vi "Add Implementations to Tree.vi"(8 "error in (no error)":errorcluster, 9 "Wired-in Class Refnum":refnum<vi>, 10 "Method Name":string, 11 "Tree Refnum":refnum<vi>) -> (0 "error out":errorcluster, 2 "Tree Refnum out":refnum<vi>, 3 "All Classes":refnum<vi>[](array[refnum]), 5 "Implementor Lookup":map{string, string}(c390))   [LabVIEW 2020, in "Peek Window.lvlib"]
uses:
  Peek Window.lvlib
  Implementor Tree Item Info.ctl
  Symbols Enum.ctl
  b7fde728-2108-4602-8341-146d6e5bbae3.vi
  <vilib>/Comparison/Equal/Equal Functor/Equal Functor.lvclass
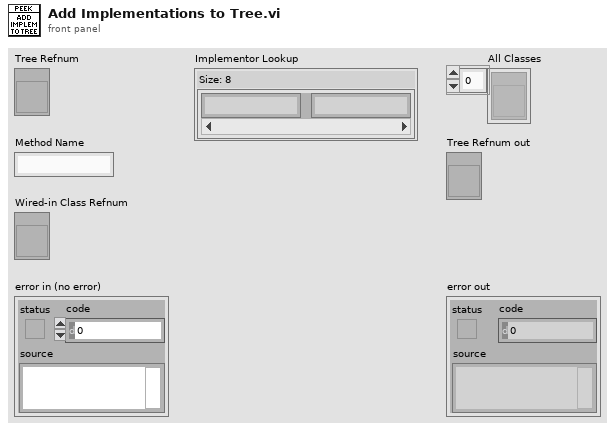
[diagram p1: front panel]
types:
  T1 = typedef "Peek Window.lvlib/Symbols Enum.ctl" = enum16{"<Blank>", "Below Here Glyph", "VI", "Dynamic Dispatch VI"}
  T2 = typedef "Peek Window.lvlib/Implementor Tree Item Info.ctl" = cluster{"ClassRef":refnum<vi>, "Implementor?":bool, "Parent ItemID":string, "Full Qualified Name":string}
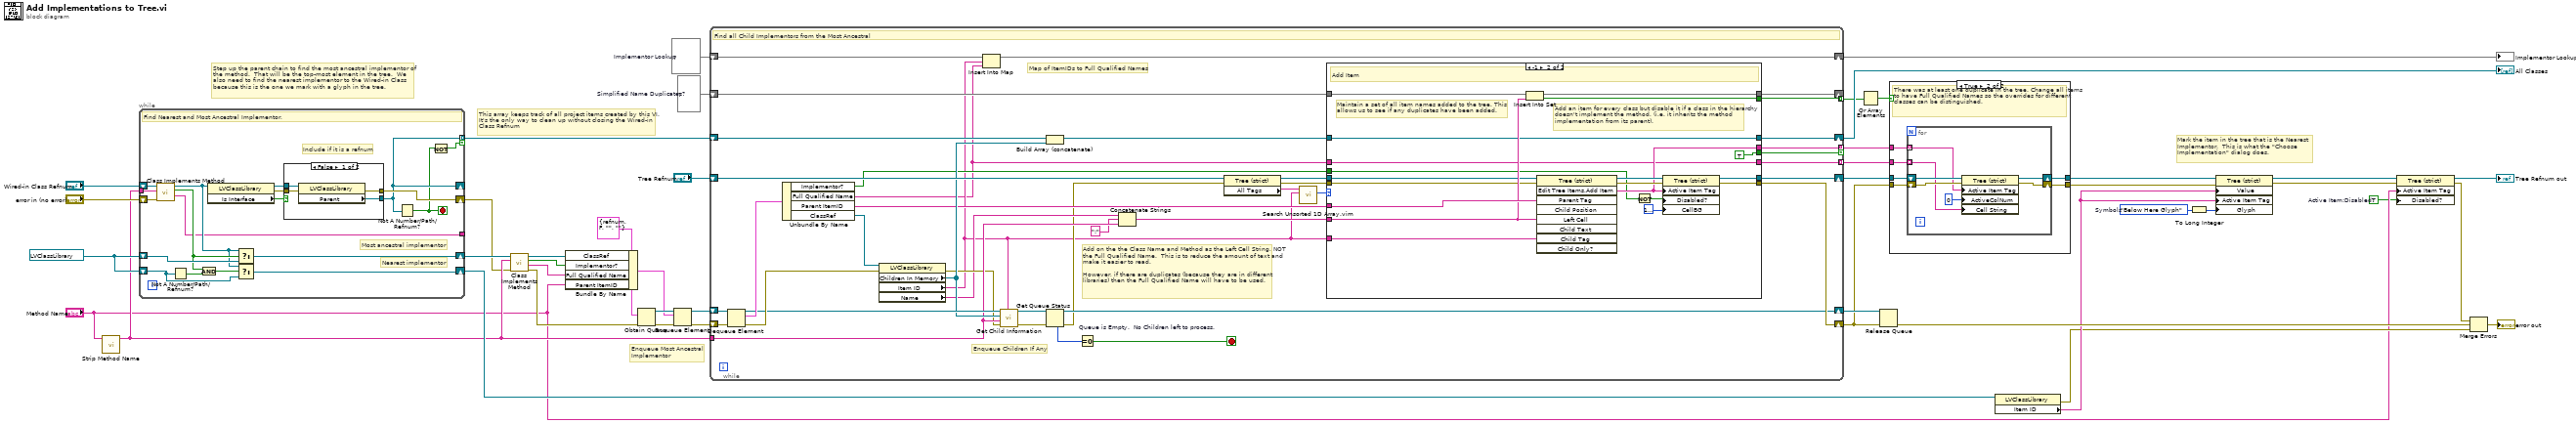
[diagram p0: block diagram]
diagram:
  w3 = TRUE  # Active Item:Disabled?
  w19 = Symbols_Enum."Below Here Glyph"  # Symbols
  w20 = set{string} {}  # Simplified Name Duplicates?
  w23 = map{string, string} {}  # Implementor Lookup
  w35 = refnum<vi> refnum ("Class Refnum out")
  w39 = T2 {"ClassRef"=refnum, "Implementor?"=FALSE, "Parent ItemID"="", "Full Qualified Name"=""} ("Cluster")
  # "Mark the item in the tree that is the Nearest Implementor.  This is what the \"Choose Implementation\" dialog does."
  # "Enqueue Most Ancestral\nImplementor"
  # "This array keeps track of all project items created by this VI.\nIt's the only way to clean up without closing the Wired-in \nClass Refnum"
  # "Step up the parent chain to find the most ancestral implementor of\nthe method.  That will be the top-most element in the tree.  We\nalso need to find the nearest implementor to the Wired-in Class\nbecause this is the one we mark with a glyph in the tree."
  n1 = call "Strip Method Name.vi"("Full Qualified Name in"="Method Name") -> ("Plain Method Name out"=w21:string)  [unwired: 10 in]
  n2 = while {
    shift-right: [w59] -> w24
    shift-left: w35 -> [w60]
    shift-right: [w47] -> _
    shift-left: "Wired-in Class Refnum" -> [w62]
    shift-right: [w53] -> w13
    shift-left: "error in (no error)" -> [w63]
    tunnel: w21 -> [w61]
    shift-right: [w54] -> w36
    shift-left: w35 -> [w55]
    tunnel: [w48] -> _
    tunnel: [w47] -> w25 mode=indexing if=w45
    stop <- w46 stop-if-true
    # "Include if it is a refnum"
    # "Nearest implementor"
    # "Most ancestral implementor"
    # "Find Nearest and Most Ancestral Implementor,"
    n3 = call "Class Implements Method.vi"("error in (no error)"=w63, "Method Name"=w61, "Class Refnum"=w62) -> ("VI Qualified Name"=w48:string, "Implements method?"=w57:bool, "Class Refnum out"=w50:refnum<vi>)  [unwired: 5 in, 1 out]
    n4 = Not A Number/Path/Refnum?(number/path/refnum=w55) -> (NaN/Path/Refnum?=w58:bool)
    n5 = And(x=w57, y=w58) -> (x .and. y?=w56:bool)
    n6 = property class="LVClassLibrary"(reference=w50) -> (reference out=w52:refnum<vi>, error out=w51:errorcluster, "Is Interface"=w49:bool)  [unwired: 1 in]
    n7 = Select(t=w50, s=w57, f=w60) -> (s? t:f=w59:refnum<vi>)
    n8 = Select(t=w50, s=w56, f=w55) -> (s? t:f=w54:refnum<vi>)
    n9 = case shown="False" w49 {
      tunnel: [w67 w68] -> w53
      tunnel: [w66 _] -> w47
      tunnel: w52 -> [w65 _]
      tunnel: w51 -> [w64 w68]
      frame False {
        n10 = property class="LVClassLibrary"(reference=w65, error in=w64) -> (error out=w67:errorcluster, "Parent"=w66:refnum<vi>)  [unwired: 1 out]
      }
      frame True {
      }
    }
    n11 = Not A Number/Path/Refnum?(number/path/refnum=w47) -> (NaN/Path/Refnum?=w46:bool)
    n12 = Not(x=w46) -> (.not. x?=w45:bool)
  }
  n13 = call "Class Implements Method.vi"("error in (no error)"=w13, "Method Name"=w21, "Class Refnum"=w24) -> ("error out"=w12:errorcluster, "VI Qualified Name"=w11:string, "Implements method?"=w10:bool, "Class Refnum out"=w7:refnum<vi>)  [unwired: 5 in]
  n14 = Bundle By Name(cluster=w39, "ClassRef"=w7, "Implementor?"=w10, "Full Qualified Name"=w11, "Parent ItemID"="Method Name") -> (w42:T2)
  n15 = Obtain Queue(element data type=w39, error in (no error)=w12) -> (queue out=w44:refnum<queue>, error out=w43:errorcluster)  [unwired: 3 in, 1 out]
  n16 = Enqueue Element(queue=w44, element=w42, error in (no error)=w43) -> (queue out=w41:refnum<queue>, error out=w40:errorcluster)  [unwired: 1 in, 1 out]
  n17 = while {
    shift-right: [w99] -> w14
    shift-left: w40 -> [w107]
    tunnel: w21 -> [w94]
    shift-right: [w72] -> w33
    shift-left: w25 -> [w97]
    tunnel: [w95] -> w29 mode=indexing if=w76
    tunnel: [w69] -> w28 mode=indexing
    tunnel: [w84] -> w32 mode=indexing
    shift-right: [w87] -> w22
    shift-left: w23 -> [w88]
    shift-right: [w85] -> _
    shift-left: w20 -> [w86]
    shift-right: [w98] -> w30
    shift-left: "Tree Refnum" -> [w100]
    shift-right: [w92] -> w38
    shift-left: w41 -> [w108]
    stop <- w106 stop-if-true
    # "Add on the the Class Name and Method as the Left Cell String, NOT the Full Qualified Name.  This is to reduce the amount of text and make it easier to read.\n\nHowever, if there are duplicates (because they are in different libraries) then the Full Qualified Name will have to be used."
    # "Enqueue Children If Any"
    # "Map of ItemIDs to Full Qualified Names"
    # "Find all Child Implementors from the Most Ancestral"
    n18 = Dequeue Element(queue=w108, error in (no error)=w107) -> (queue out=w102:refnum<queue>, element=w104:T2, error out=w103:errorcluster)  [unwired: 1 in, 1 out]
    n19 = Unbundle By Name(w104) -> ("Implementor?"=w81:bool, "Full Qualified Name"=w70:string, "Parent ItemID"=w90:string, "ClassRef"=w82:refnum<vi>)
    n20 = property class="LVClassLibrary"(reference=w82, error in=w103) -> (error out=w91:errorcluster, "Children In Memory"=w96:refnum<vi>[], "Item ID"=w74:string, "Name"=w80:string)  [unwired: 1 out]
    n21 = Insert Into Map(map in=w88, key=w74, value=w70) -> (map out=w87:map{string, string})  [unwired: 2 out]
    n22 = call "Get Child Information.vi"("ParentID"=w74, "error in (no error)"=w91, "Plain Method Name in"=w94, "Children in Memory"=w96, "Queue in"=w102) -> ("error out"=w89:errorcluster, "Queue out"=w101:refnum<queue>)  [unwired: 5 in]
    n23 = Build Array (concatenate)(w97, w96) -> (w71:refnum<vi>[])
    n24 = Get Queue Status(queue=w101, error in (no error)=w89) -> (queue out=w92:refnum<queue>, error out=w78:errorcluster, # elements in queue=w105:i32)  [unwired: 1 in, 5 out]
    n25 = Equal To 0? "Queue is Empty.  No Children left to process."(x=w105) -> (x = 0?=w106:bool)
    n26 = Concatenate Strings(w80, ":" ("element"), w94) -> (w83:string)
    n27 = property class="Tree (strict)"(reference=w100, error in=w78) -> (reference out=w79:refnum<vi>, error out=w77:errorcluster, "All Tags"=w75:string[])
    n28 = call "Search Unsorted 1D Array.vim"("element"=w74, "unsorted 1D array"=w75) -> ("index of element"=w73:i32)  [unwired: 9 in]
    n29 = case shown="-1" w73 {
      tunnel: [w111 w129] -> w99
      tunnel: [w112 w128] -> w98
      tunnel: [_ w127] -> w95
      tunnel: w90 -> [_ w126]
      tunnel: w86 -> [w113 w125]
      tunnel: [w113 w124] -> w85
      tunnel: [_ w123] -> w84
      tunnel: w83 -> [_ w122]
      tunnel: w81 -> [_ w121]
      tunnel: w74 -> [_ w120]
      tunnel: w79 -> [w112 w119]
      tunnel: w77 -> [w111 w118]
      tunnel: [_ TRUE] -> w76
      tunnel: [w110 w116] -> w72
      tunnel: w71 -> [w110 w116]
      tunnel: w70 -> [w109 w115]
      tunnel: [w109 w115] -> w69
      frame Default {
        # "Duplicate Tag. Ignore Item."
      }
      frame -1 {
        # "Add an item for every class but disable it if a class in the hierarchy doesn't implement the method, (i.e. it inherits the method implementation from its parent)."
        # "Maintain a set of all item names added to the tree. This allows us to see if any duplicates have been added."
        # "Add Item"
        n30 = Insert Into Set(10:w122, 11:w125) -> (2:w123:bool, 3:w124:set{string})
        n31 = invoke class="Tree (strict)" method="Edit Tree Items.Add Item"(reference=w119, error in=w118, "Parent Tag"=w126, "Left Cell"=w122, "Child Tag"=w120) -> (reference out=w132:refnum<vi>, error out=w131:errorcluster, "Edit Tree Items:Add Item"=w127:string)  [unwired: 4 in, 6 out]
        n32 = Not(x=w121) -> (.not. x?=w130:bool)
        n33 = property class="Tree (strict)"(reference=w132, error in=w131, "Active Item Tag"=w127, "Disabled?"=w130, "CellBG"=u32 16777238) -> (reference out=w128:refnum<vi>, error out=w129:errorcluster)
      }
    }
  }
  "All Classes" <- w33
  "Implementor Lookup" <- w22
  n34 = Or Array Elements(Boolean array=w32) -> (logical OR=w31:bool)
  n35 = Release Queue(queue=w38, error in (no error)=w14) -> (error out=w34:errorcluster)  [unwired: 1 in, 2 out]
  n36 = case shown="True" w31 {
    tunnel: w30 -> [w134 w138]
    tunnel: [w134 w137] -> w18
    tunnel: w14 -> [w133 w136]
    tunnel: [w133 w135] -> w9
    tunnel: w29 -> [_ w140]
    tunnel: w28 -> [_ w139]
    frame False {
      # "No duplicate items in the tree, no need to update class file names in the tree to qualified class names."
    }
    frame True {
      # "There was at least one duplicate in the tree. Change all items to have Full Qualified Names so the overrides for different classes can be distinguished."
      n37 = for {
        tunnel: w140 -> [w143] mode=indexing
        tunnel: w139 -> [w141] mode=indexing
        shift-right: [w146] -> w137
        shift-left: w138 -> [w147]
        shift-right: [w144] -> w135
        shift-left: w136 -> [w145]
        n38 = property class="Tree (strict)"(reference=w147, error in=w145, "Active Item Tag"=w143, "ActiveColNum"=0 ("Active Cell:Active Column Number"), "Cell String"=w141) -> (reference out=w146:refnum<vi>, error out=w144:errorcluster)
      }
    }
  }
  n39 = property class="LVClassLibrary"(reference=w36) -> (error out=w8:errorcluster, "Item ID"=w17:string)  [unwired: 1 in, 1 out]
  n40 = To Long Integer(number=w19) -> (32bit integer=w15:i32)
  n41 = property class="Tree (strict)"(reference=w18, error in=w9, "Value"=w17, "Active Item Tag"=w17, "Glyph"=w15) -> (reference out=w6:refnum<vi>, error out=w2:errorcluster)
  n42 = property class="Tree (strict)"(reference=w6, error in=w2, "Active Item Tag"="Method Name", "Disabled?"=w3) -> (reference out=→"Tree Refnum out":refnum<vi>, error out=w1:errorcluster)
  n43 = Merge Errors(w1, w34, w8) -> (→"error out":errorcluster)
